vi "GetIOVariable.vi"(8 "error in (no error)":errorcluster, 10 "Channel Number":i32, 11 "IO Ref":refnum<k21>) -> (0 "error out":errorcluster, 2 "Type":T1, 3 "IO Variable Ref":refnum<k21>)   [LabVIEW 2017, in "ScanEngine.lvlib"]
uses:
  <vilib>/addons/InsightCM/Devices/Shared/Common/ScanEngine/ScanEngine.lvlib
  <vilib>/Utility/Data Type/Type Definitions/Data Type.ctl
  <resource>/objmgr/cRIO.rc
  <resource>/objmgr/ni.var.rc
  <vilib>/Utility/Data Type/NI_Data Type.lvlib
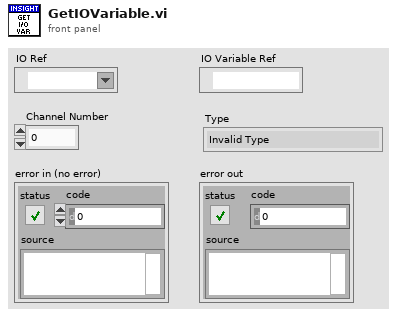
[diagram p1: front panel]
types:
  T1 = typedef "NI_Data Type.lvlib/Data Type.ctl" = enum8{"Invalid Type", "Void", "I8", "I16", "I32", "I64", "U8", "U16", "U32", "U64", "Single Float", "Double Float", "Extended Float", "Single Complex", "Double Complex", "Extended Complex", "Enum U8", "Enum U16", "Enum U32", "Enum U64", "Single Float With Unit", "Double Float With Unit", "Extended Float With Unit", "Single Complex with Unit", "Double Complex with Unit", "Extended Complex with Unit", "Boolean", "String", "Path", "Picture", "Tag", "Array", "Cluster", "Variant", "LV Variant", "Waveform", "Timestamp", "Digital Waveform", "Digital Data", "ExpressData", "Refnum", "External Data", "VI", "Poly VI", "LabVIEW Class Instance", "Fixed Point"}
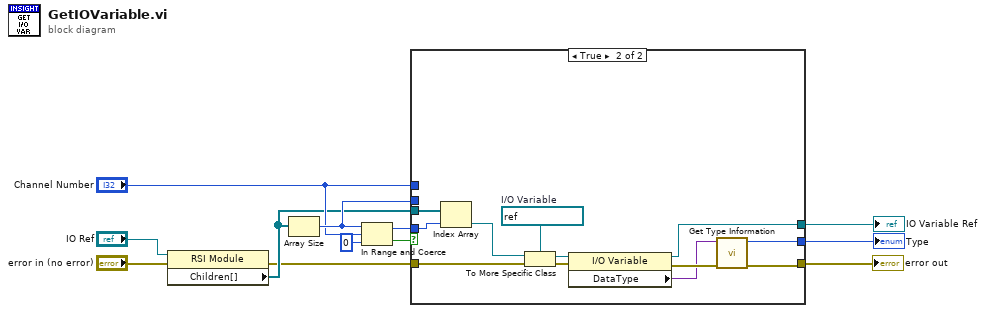
[diagram p0: block diagram]
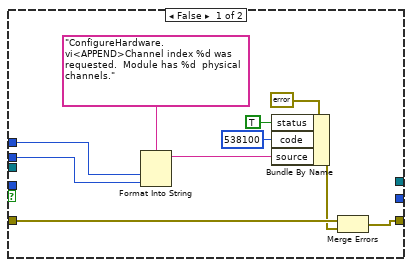
[diagram p2: hidden frame]
diagram:
  n1 = property class="RSI Module"(reference="IO Ref", error in="error in (no error)") -> (error out=w2:errorcluster, "Children[]"=w7:refnum<k21>[])  [unwired: 1 out]
  n2 = Array Size(array=w7) -> (size(s)=w10:i32)
  n3 = In Range and Coerce(upper limit=w10, x="Channel Number", lower limit=0) -> (coerced(x)=w6:i32, In Range?=w8:bool)
  n4 = case shown="True" w8 {
    tunnel: w2 -> [w17 w32]
    tunnel: [w16 w23] -> w11
    tunnel: [_ w27] -> w12
    tunnel: w6 -> [_ w31]
    tunnel: w7 -> [_ w30]
    tunnel: "Channel Number" -> [w14 _]
    tunnel: w10 -> [w15 _]
    tunnel: [_ w24] -> w1
    frame False {
      n5 = Format Into String(format string="ConfigureHardware.vi<APPEND>Channel index %d was requested.  Module has %d  physical channels.", w14, w15) -> (resulting string=w20:string)  [unwired: 2 in, 1 out]
      n6 = Bundle By Name(cluster=errorcluster {"status"=TRUE, "code"=538100, "source"=""} ("error in"), "status"=TRUE, "code"=538100, "source"=w20) -> (w13:errorcluster)
      n7 = Merge Errors(w17, w13) -> (w16:errorcluster)
    }
    frame True {
      w34 = refnum<k21> refnum  # I/O Variable
      n8 = Index Array(array=w30, index=w31) -> (element=w33:refnum<k21>)
      n9 = To More Specific Class(target class=w34, reference=w33, error in=w32) -> (specific class reference=w28:refnum<k21>, error out=w29:errorcluster)
      n10 = property class="I/O Variable"(reference=w28, error in=w29) -> (reference out=w27:refnum<k21>, error out=w26:errorcluster, "DataType"=w25:variant)
      n11 = call <vilib>:"Get Type Information.vi"("error in (no error)"=w26, "Variant"=w25) -> ("error out"=w23:errorcluster, "Type"=w24:T1)  [unwired: 5 in, 3 out]
    }
  }
  "IO Variable Ref" <- w12
  "error out" <- w11
  "Type" <- w1
